vi "subDefaultImage.vi"(2 "error in (no error)":errorcluster) -> (0 "error out":errorcluster, 3 "Image":T1(plugin-control))   [LabVIEW 2017]
panel:
  # "This VI processes an image for display from\na relative path location."
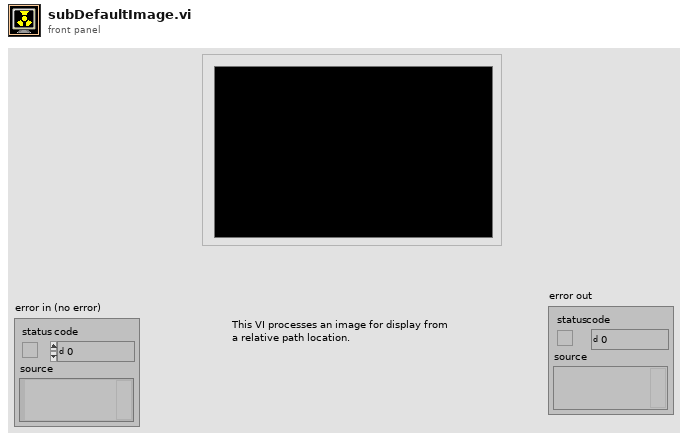
[diagram p1: front panel]
types:
  T1 = typedef "IMAQ Image.ctl" = refnum<image>
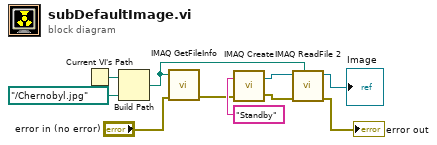
[diagram p0: block diagram]
diagram:
  n1 = Current VI's Path() -> (path=w7:path)
  n2 = Build Path(base path=w7, name or relative path=path "../Chernobyl.jpg") -> (appended path=w6:path)
  n3 = call "IMAQ GetFileInfo"("error in (no error)"="error in (no error)", "File Path"=w6) -> ("error out"=w3:errorcluster)  [unwired: 3 in, 6 out]
  n4 = call "IMAQ Create"("Image Name"="Standby" ("name or relative path"), "error in (no error)"=w3) -> ("New Image"=w10:T1, "error out"=w2:errorcluster)  [unwired: 3 in]
  n5 = call "IMAQ ReadFile 2"("File Path"=w6, "error in (no error)"=w2, "Image"=w10) -> ("error out"=→"error out":errorcluster, "Image Out"=→"Image":T1)  [unwired: 4 in, 3 out]
